vi "TCP Listener.vi"(8 "error in":errorcluster) -> (0 "error out":errorcluster, 3 "Port Config":T1)   [LabVIEW 2022 SP3]
uses:
  <vilib>/Utility/file.llb/Read Delimited Spreadsheet (DBL).vi
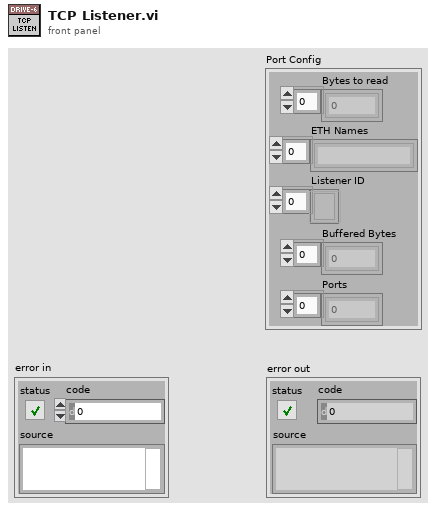
[diagram p1: front panel]
types:
  T1 = cluster{"Bytes to read":i32[], "ETH Names":string[], "Listener ID":refnum<k5>[], "Buffered Bytes":i32[], "Ports":u16[]}
  T2 = typedef "D6 Root path.ctl" = cluster{"Data":path, "Sub VI's":path, "Source code":path}
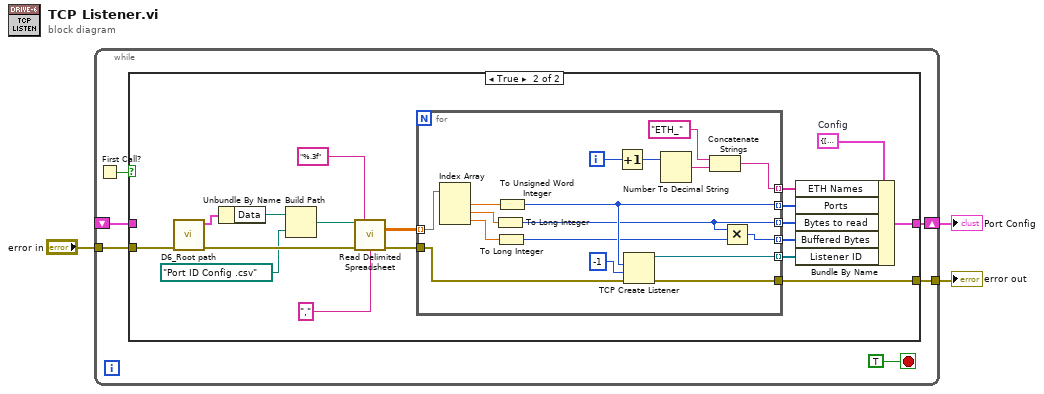
[diagram p0: block diagram]
diagram:
  n1 = while {
    tunnel: "error in" -> [w8]
    shift-right: [w7] -> w2
    shift-left: _ -> [w5]
    tunnel: [w4] -> w1
    stop <- TRUE stop-if-true
    n2 = First Call?() -> (First Call?: T/F=w9:bool)
    n3 = case shown="True" w9 {
      tunnel: w8 -> [w10 w19]
      tunnel: [w11 w21] -> w7
      tunnel: w5 -> [w11 _]
      tunnel: [w10 w20] -> w4
      frame False {
      }
      frame True {
        w27 = T1 {"Bytes to read"=[], "ETH Names"=[], "Listener ID"=[], "Buffered Bytes"=[], "Ports"=[]}  # Config
        n4 = call "D6_Root path.vi"("error in (no error)"=w19) -> ("error out"=w14:errorcluster, "Root Path"=w16:T2)  [unwired: 9 in]
        n5 = Unbundle By Name(w16) -> ("Data"=w15:path)
        n6 = Build Path(base path=w15, name or relative path=path "Port ID Config .csv") -> (appended path=w13:path)
        n7 = call-poly <vilib>:"Read Delimited Spreadsheet.vi"("file path (dialog if empty)"=w13, "format (%.3f)"="%.3f", "error in (no error)"=w14, "delimiter (\\t)"="," ("delimiter (\\t)")) -> ("all rows"=w29:dbl[][], "error out"=w28:errorcluster)  [unwired: 6 in, 4 out]
        n8 = for {
          tunnel: w29 -> [w46] mode=indexing
          tunnel: w28 -> [w34]
          tunnel: [w40] -> w26 mode=indexing
          tunnel: [w39] -> w25 mode=indexing
          tunnel: [w31] -> w24 mode=indexing
          tunnel: [w32] -> w23 mode=indexing
          tunnel: [w36] -> w22 mode=indexing
          tunnel: [w33] -> w20
          i -> [w42]
          n9 = Index Array(array=w46) -> (element #1=w41:dbl, element #2=w38:dbl, element #3=w37:dbl)  [unwired: 3 in]
          n10 = To Long Integer(number=w38) -> (32bit integer=w31:i32)
          n11 = To Long Integer(number=w37) -> (32bit integer=w30:i32)
          n12 = To Unsigned Word Integer(number=w41) -> (unsigned 16bit integer=w40:u16)
          n13 = Increment(x=w42) -> (x+1=w45:i32)
          n14 = TCP Create Listener(8:w34, 9:-1 ("timeout ms (25000)"), 10:w40) -> (0:w33:errorcluster, 3:w36:refnum<k5>)  [unwired: 2 in, 1 out]
          n15 = Number To Decimal String(number=w45) -> (decimal integer string=w44:string)  [unwired: 1 in]
          n16 = Concatenate Strings("ETH_", w44) -> (w39:string)
          n17 = Multiply(x=w31, y=w30) -> (x*y=w32:i32)
        }
        n18 = Bundle By Name(cluster=w27, "ETH Names"=w25, "Ports"=w26, "Bytes to read"=w24, "Buffered Bytes"=w23, "Listener ID"=w22) -> (w21:T1)
      }
    }
  }
  "Port Config" <- w2
  "error out" <- w1
